vi "Частотный анализ текста.vi"() -> ()   [LabVIEW 2018]
panel:
  out "Частота букв":cluster{dbl, "Алфавит out":string}[](array[cluster]) {"?" scale=0.0..14.0}
  in  "Язык":enum16{"Русский", "Английский"}(ring)
  in  "Табличка":i32(listbox)
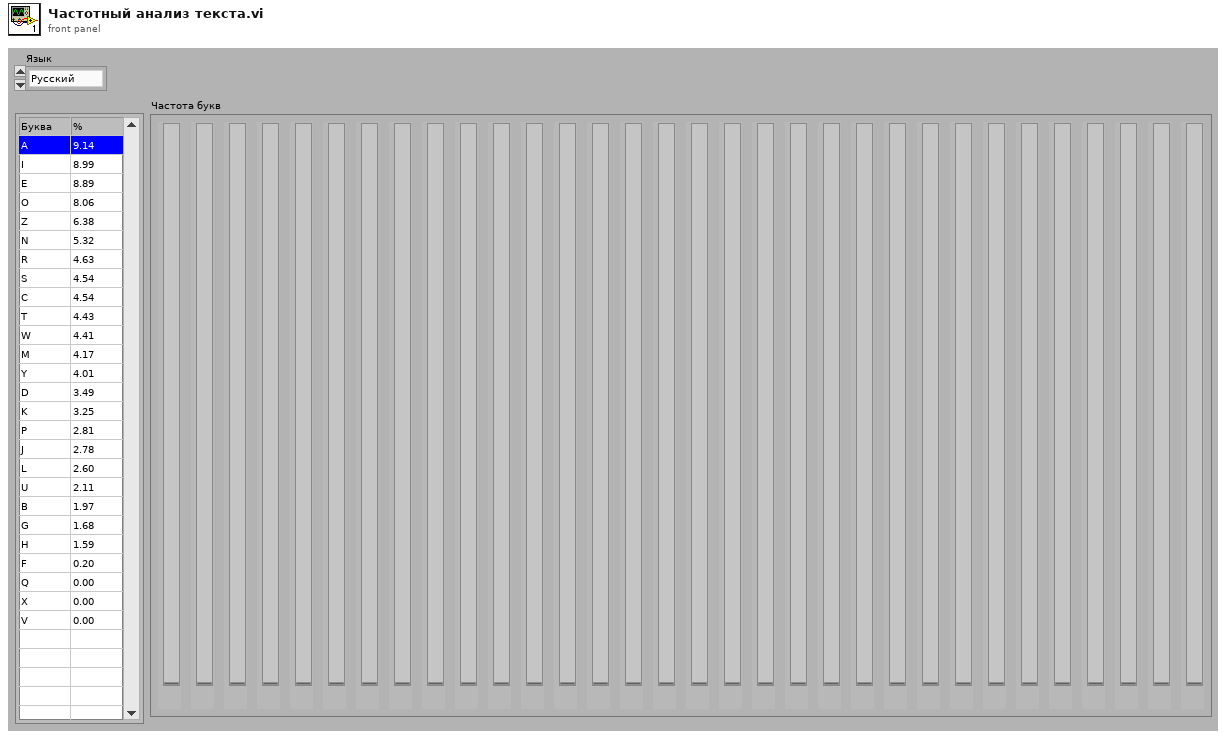
[diagram p1: front panel]
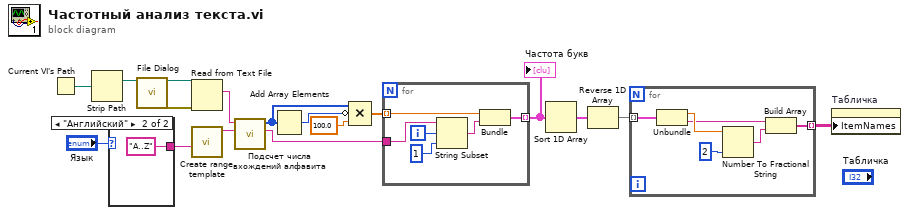
[diagram p0: block diagram]
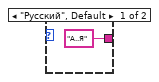
[diagram p2: hidden frame]
diagram:
  n1 = Current VI's Path() -> (path=w4:path)
  n2 = Strip Path(path=w4) -> (stripped path=w1:path)  [unwired: 1 out]
  n3 = case shown="\"Английский\"" "Язык" {
    tunnel: ["А..Я" ("Range Template (А..Я)") "A..Z" ("Range Template (А..Я)")] -> w15
    frame "Русский", Default {
    }
    frame "Английский" {
    }
  }
  n4 = call "File Dialog"("start path"=w1) -> ("selected path"=w3:path, "error out"=w2:errorcluster)  [unwired: 11 in, 2 out]
  n5 = Read from Text File(file (use dialog)=w3, error in=w2) -> (text=w17:string)  [unwired: 2 in, 3 out]
  n6 = call "Create range template.vi"("Range Template (А..Я)"=w15) -> ("Template String"=w14:string)  [unwired: 7 in, 3 out]
  n7 = call "Подсчет числа вхождений алфавита.vi"("Алфавит"=w14, "Текст"=w17) -> ("Алфавит out"=w13:string, "Число вхождений"=w8:i32[])  [unwired: 8 in]
  n8 = Add Array Elements(numeric array=w8) -> (sum=w7:i32)
  n9 = Compound Arithmetic op=MULTIPLY(w8, invert w7, 100.0) -> (w5:dbl[])
  n10 = for {
    tunnel: w5 -> [w25] mode=indexing
    tunnel: w13 -> [w22]
    tunnel: [w24] -> w11 mode=indexing
    i -> [w21]
    n11 = String Subset(string=w22, offset (0)=w21, length (rest)=1 ("length (rest)")) -> (substring=w20:string)
    n12 = Bundle(w25, "Алфавит out"=w20) -> (w24:cluster{dbl, "Алфавит out":string})  [unwired: 1 in]
  }
  "Частота букв" <- w11
  n13 = Sort 1D Array(array=w11) -> (sorted array=w12:cluster{dbl, "Алфавит out":string}[])
  n14 = Reverse 1D Array(array=w12) -> (reversed array=w10:cluster{dbl, "Алфавит out":string}[])
  n15 = for {
    tunnel: w10 -> [w31] mode=indexing
    tunnel: [w26] -> w9 mode=indexing
    n16 = Unbundle(w31) -> (w30:dbl, "Алфавит out"=w28:string)
    n17 = Number To Fractional String(number=w30, precision (6)=i16 2) -> (F-format string=w27:string)  [unwired: 2 in]
    n18 = Build Array(w28, w27) -> (w26:string[])
  }
  n19 = property on="Табличка" class="MCListbox (strict)"("ItemNames"=w9) -> ()  [unwired: 2 in, 2 out]
